vi "Find Terminations.vi"(0 "State in":refnum<class "State.lvclass">, 7 "Type":T1, 11 "error in (no error)":errorcluster) -> (4 "State thru":refnum<class "State.lvclass">, 8 "Terminations":refnum<class "Termination.lvclass">[](array[class]), 15 "error out":errorcluster)   [LabVIEW 2020, in "State.lvclass"]
uses:
  State.lvclass
  Typedefs/Tosca-Event Type.ctl
  Termination/Termination.lvclass
  State.lvclass/State.ctl
  Termination/Termination.lvclass/Termination.ctl
  Termination/Read Type.vi
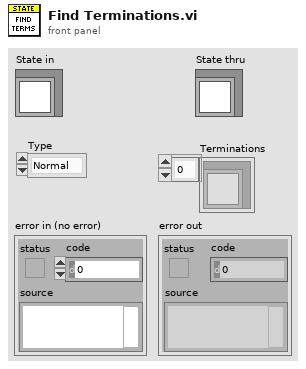
[diagram p1: front panel]
types:
  T1 = typedef "Tosca-Event Type.ctl" = enum16{"Normal", "CS+", "CS-"}
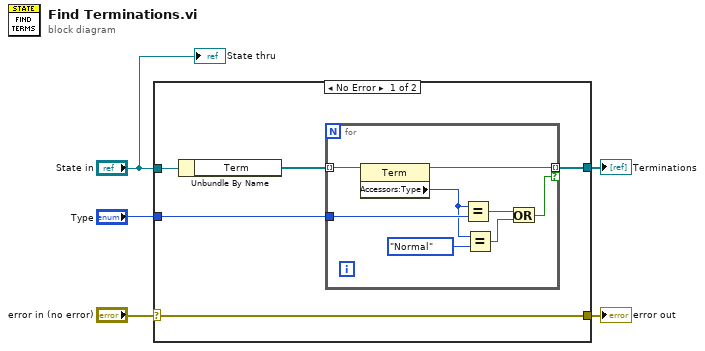
[diagram p0: block diagram]
diagram:
  n1 = case shown="No Error" "error in (no error)" {
    selector: "error in (no error)" -> [w10 w19]
    tunnel: [w10 w19] -> w4
    tunnel: "State in" -> [w9 _]
    tunnel: "Type" -> [w8 _]
    tunnel: [w6 _] -> w1
    frame No Error {
      n2 = Unbundle By Name(w9) -> ("Term"=w7:refnum<class "Termination.lvclass">[])
      n3 = for {
        tunnel: w7 -> [w18] mode=indexing
        tunnel: w8 -> [w17]
        tunnel: [w16] -> w6 mode=indexing if=w14
        n4 = property class="Term"(reference=w18) -> (reference out=w16:refnum<class "Termination.lvclass">, "Accessors:Type"=w13:T1)  [unwired: 1 in, 1 out]
        n5 = Equal?(x=w13, y=w17) -> (x = y?=w15:bool)
        n6 = Equal?(x=w13, y=Tosca-Event_Type."Normal") -> (x = y?=w11:bool)
        n7 = Or(x=w15, y=w11) -> (x .or. y?=w14:bool)
      }
    }
    frame Error {
    }
  }
  "error out" <- w4
  "Terminations" <- w1
  "State thru" <- "State in"
